vi "Excel_Set_Chart_Axis_Font.vi"(0 "Excel._Worksheet":refnum<k7>, 1 "Shapes":refnum<k7>, 5 "type":i32(ring)=1 items=["xlCategory"=1, "xlSeriesAxis"=3, "xlValue"=2], 7 "number format":string, 9 "Chart index":i16=-1, 11 "error in (no error)":errorcluster, 12 "axis font":T1={"font style"="", "bold"=FALSE, "italic"=FALSE, "underline"=FALSE, "size"=10.0, "color"=-16777216} {"color" items=["wdColorAutomatic"=-16777216, "wdColorBlack"=0, "wdColorBlue"=16711680, "wdColorTurquoise"=16776960, "wdColorBrightGreen"=65280, "wdColorPink"=16711935, "wdColorRed"=255, "wdColorYellow"=65535, "wdColorWhite"=16777215, "wdColorDarkBlue"=8388608, "wdColorTeal"=8421376, "wdColorGreen"=32768, "wdColorViolet"=8388736, "wdColorDarkRed"=128, "wdColorDarkYellow"=32896, "wdColorBrown"=13209, "wdColorOliveGreen"=13107, "wdColorDarkGreen"=13056, "wdColorDarkTeal"=6697728, "wdColorIndigo"=10040115, "wdColorOrange"=26367, "wdColorBlueGray"=10053222, "wdColorLightOrange"=39423, "wdColorLime"=52377, "wdColorSeaGreen"=6723891, "wdColorAqua"=13421619, "wdColorLightBlue"=16737843, "wdColorGold"=52479, "wdColorSkyBlue"=16763904, "wdColorPlum"=6697881, "wdColorRose"=13408767, "wdColorTan"=10079487, "wdColorLightYellow"=10092543, "wdColorLightGreen"=13434828, "wdColorLightTurquoise"=16777164, "wdColorPaleBlue"=16764057, "wdColorLavender"=16751052, "wdColorGray05"=15987699, "wdColorGray10"=15132390, "wdColorGray125"=14737632, "wdColorGray15"=14277081, "wdColorGray20"=13421772, "wdColorGray25"=12632256, "wdColorGray30"=11776947, "wdColorGray35"=10921638, "wdColorGray375"=10526880, "wdColorGray40"=10066329, "wdColorGray45"=9211020, "wdColorGray50"=8421504, "wdColorGray55"=7566195, "wdColorGray60"=6710886, "wdColorGray625"=6316128, "wdColorGray65"=5855577, "wdColorGray70"=5000268, "wdColorGray75"=4210752, "wdColorGray80"=3355443, "wdColorGray85"=2500134, "wdColorGray875"=2105376, "wdColorGray90"=1644825, "wdColorGray95"=789516]; "size" format="%0.2f"}, 13 "title":string) -> (15 "error out":errorcluster)   [LabVIEW 2010, in "NI_ReportGenerationToolkit.lvlib"]
uses:
  <vilib>/addons/_office/NI_ReportGenerationToolkit.lvlib
panel:
  in  "Excel._OLEObject":refnum<k7>
  in  "Graph.Axes":refnum<k7>
  in  "Graph.Chart":refnum<k7>
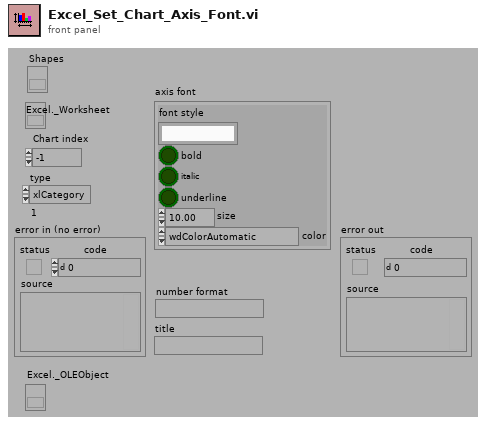
[diagram p1: front panel]
types:
  T1 = cluster{"font style":string, "bold":bool, "italic":bool, "underline":bool, "size":sgl, "color":i32}
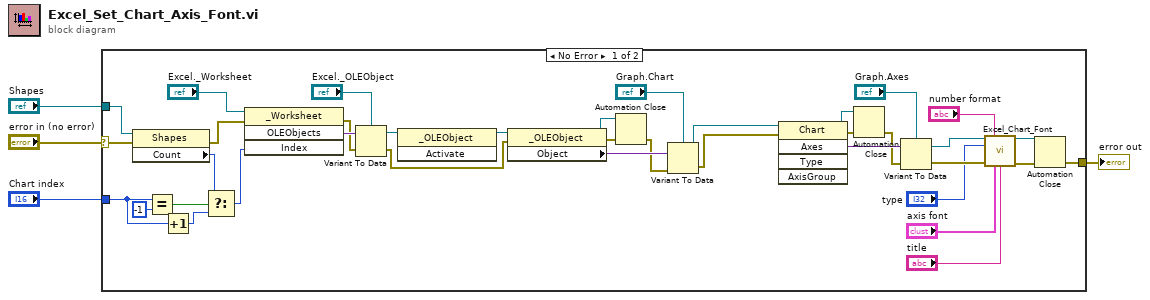
[diagram p0: block diagram]
diagram:
  n1 = case shown="No Error" "error in (no error)" {
    selector: "error in (no error)" -> [w5 w42]
    tunnel: "Chart index" -> [w31 _]
    tunnel: [w20 w42] -> w3
    tunnel: "Shapes" -> [w6 _]
    frame No Error {
      n2 = property class="Shapes"(reference=w6, error in=w5) -> (error out=w35:errorcluster, "Count"=w30:i32)  [unwired: 1 out]
      n3 = Equal?(x=w31, y=i16 -1) -> (x = y?=w34:bool)
      n4 = Increment(x=w31) -> (x+1=w32:i16)
      n5 = Select(t=w30, s=w34, f=w32) -> (s? t:f=w29:i32)
      n6 = invoke class="_Worksheet" method="OLEObjects"(reference="Excel._Worksheet", error in=w35, "Index"=w29) -> (error out=w38:errorcluster, "OLEObjects"=w39:variant)  [unwired: 1 in, 2 out]
      n7 = Variant To Data(error in=w38, Variant=w39, type="Excel._OLEObject") -> (error out=w23:errorcluster, data=w25:refnum<k7>)
      n8 = invoke class="_OLEObject" method="Activate"(reference=w25) -> (reference out=w24:refnum<k7>)  [unwired: 2 in, 2 out]
      n9 = property class="_OLEObject"(reference=w24, error in=w23) -> (reference out=w36:refnum<k7>, error out=w37:errorcluster, "Object"=w28:variant)
      n10 = Automation Close(3:w37, 5:w36) -> (0:w27:errorcluster)
      n11 = Variant To Data(error in=w27, Variant=w28, type="Graph.Chart") -> (error out=w26:errorcluster, data=w22:refnum<k7>)
      n12 = invoke class="Chart" method="Axes"(reference=w22, error in=w26) -> (reference out=w12:refnum<k7>, error out=w13:errorcluster, "Axes"=w19:variant)  [unwired: 3 in, 2 out]
      n13 = Automation Close(3:w13, 5:w12) -> (0:w15:errorcluster)
      n14 = Variant To Data(error in=w15, Variant=w19, type="Graph.Axes") -> (error out=w17:errorcluster, data=w16:refnum<k7>)
      n15 = call <vilib>:"Excel_Chart_Font.vi"("axes in"=w16, "number format"="number format", "type"="type", "error in (no error)"=w17, "axis font"="axis font", "title"="title") -> ("axes out"=w10:refnum<k7>, "error out"=w11:errorcluster)  [unwired: 4 in, 4 out]
      n16 = Automation Close(3:w11, 5:w10) -> (0:w20:errorcluster)
    }
    frame Error {
    }
  }
  "error out" <- w3
